vi "Targets 2 Command Data.vi"(6 "Combined":bool, 10 "Target  Inputs":T1[](array[typedef])) -> (2 "LBCB 2 Command Data":T3, 3 "LBCB 1 Command Data":T3)   [LabVIEW 2013]
uses:
  Target Data.ctl
  Target.ctl
  Data Access Objects/Metadata/LBCB Number.ctl
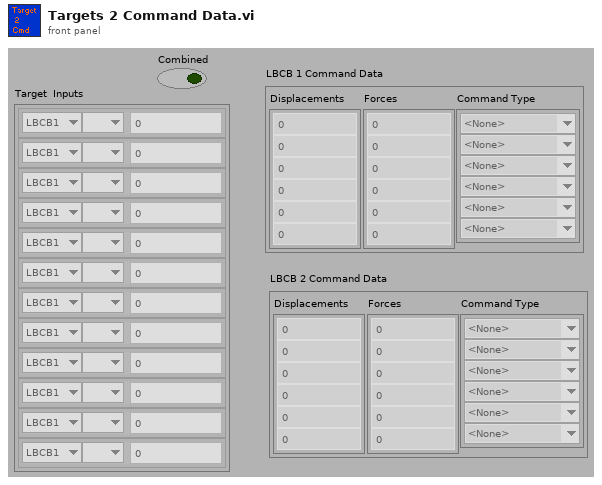
[diagram p1: front panel]
types:
  T1 = typedef "Target.ctl" = cluster{"LBCB Number":T2, "DOF Vectors":enum16{" ", "Dx", "Dy", "Dz", "Rx", "Ry", "Rz", "Fx", "Fy", "Fz", "Mx", "My", "Mz"}, "Amount":dbl}
  T2 = typedef "LBCB Number.ctl" = enum16{"LBCB1", "LBCB2"}
  T3 = typedef "Target Data.ctl" = cluster{"Displacements":dbl[], "Command Type":enum16{"<None>", "Displacement", "Force"}[], "Forces":dbl[]}
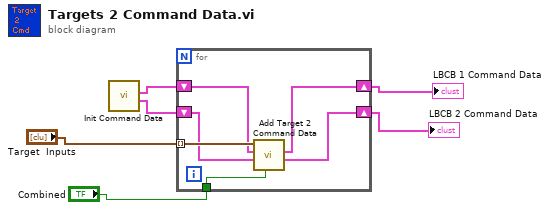
[diagram p0: block diagram]
diagram:
  n1 = call "Init Command Data.vi"() -> ("LBCB 2 Command Data"=w4:T3, "LBCB 1 Command Data"=w5:T3)  [unwired: 10 out]
  n2 = for {
    tunnel: "Target  Inputs" -> [w12] mode=indexing
    shift-right: [w9] -> w3
    shift-left: w5 -> [w10]
    shift-right: [w8] -> w2
    shift-left: w4 -> [w11]
    tunnel: "Combined" -> [w7]
    n3 = call "Add Target 2 Command Data.vi"("Combined"=w7, "LBCB 2 Command Data In"=w11, "LBCB 1 Command Data In"=w10, "Target"=w12) -> ("LBCB 2 Command Data Out"=w8:T3, "LBCB 1 Command Data Out"=w9:T3)  [unwired: 1 in, 5 out]
  }
  "LBCB 1 Command Data" <- w3
  "LBCB 2 Command Data" <- w2
